vi "运维调试.vi"() -> ()   [LabVIEW 2016]
uses:
  <vilib>/Utility/miscctls.llb/LVPointTypeDef.ctl
  PLC/PLC.lvlib
  <vilib>/Utility/config.llb/NI_LVConfig.lvlib
panel:
  in  "运维调试菜单":T1(xcontrol)
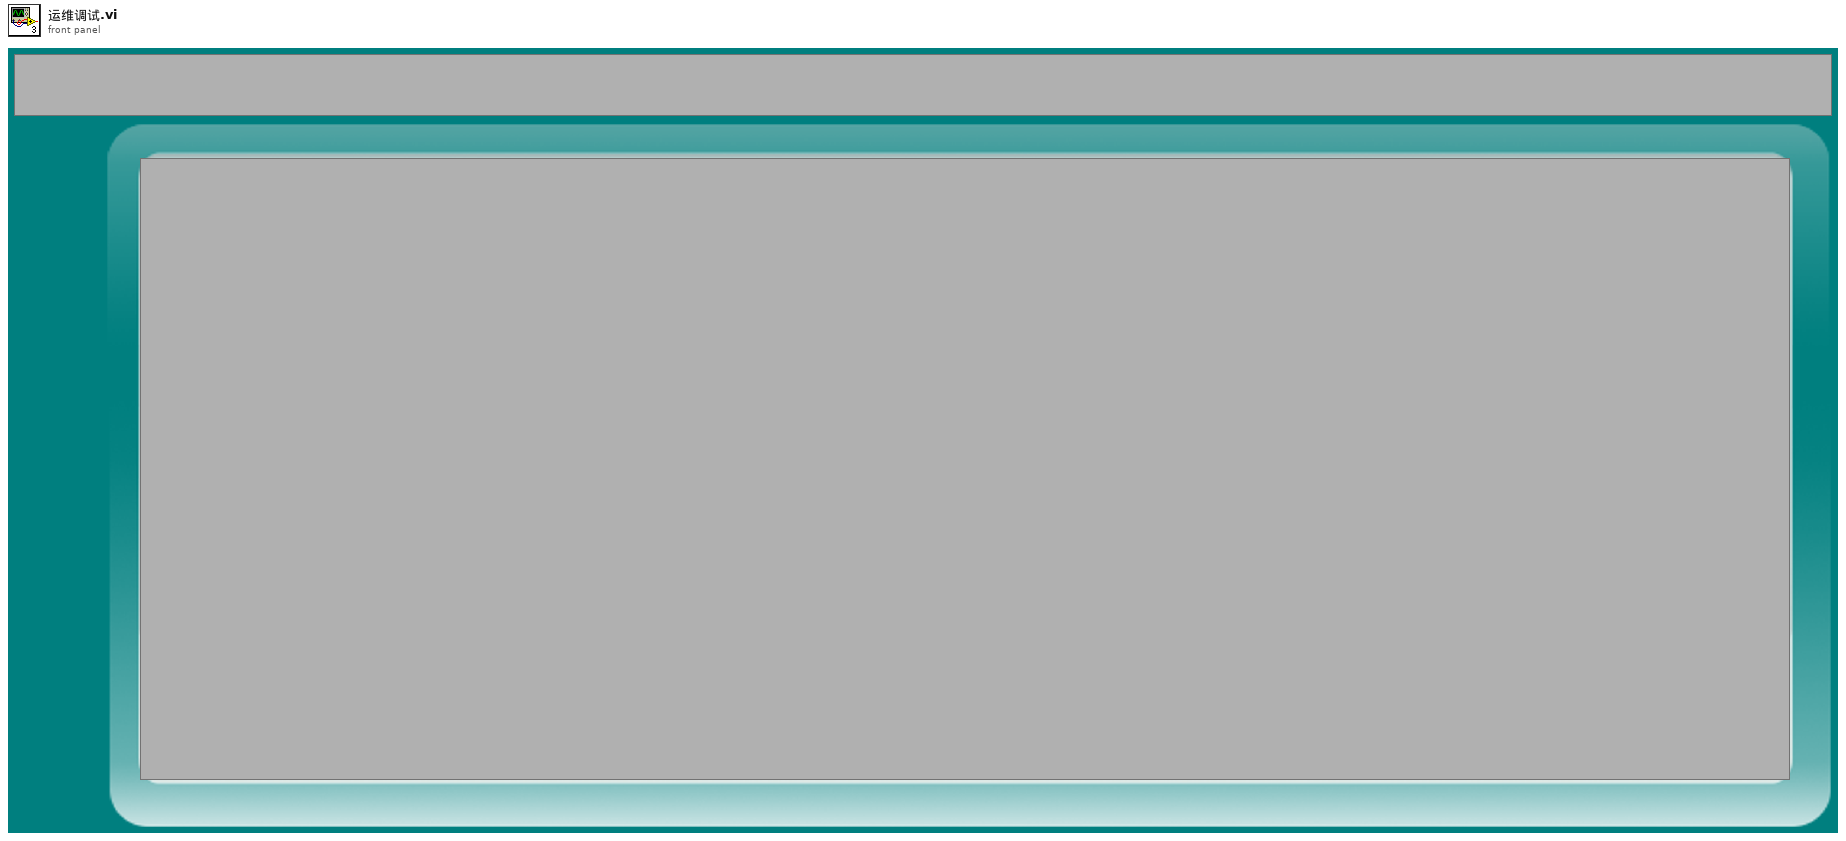
[diagram p1: front panel]
types:
  T1 = enum16{"电源管理", "采配水", "氨氮", "总磷", "总氮", "多参数", "CODMn", "CODcr", "流量计", "质控单元", "超标留样", "其他"}
  T2 = typedef "NI_LVConfig.lvlib/Config Data RefNum.ctl" = refnum<k1>
  T3 = typedef "LVPointTypeDef.ctl" = cluster{"Horizontal":i16, "Vertical":i16}
  T4 = enum16{"Enabled", "Disabled", "Disabled and Grayed Out"}
  T5 = enum32{"Bad", "Idle", "Run top level", "Running"}
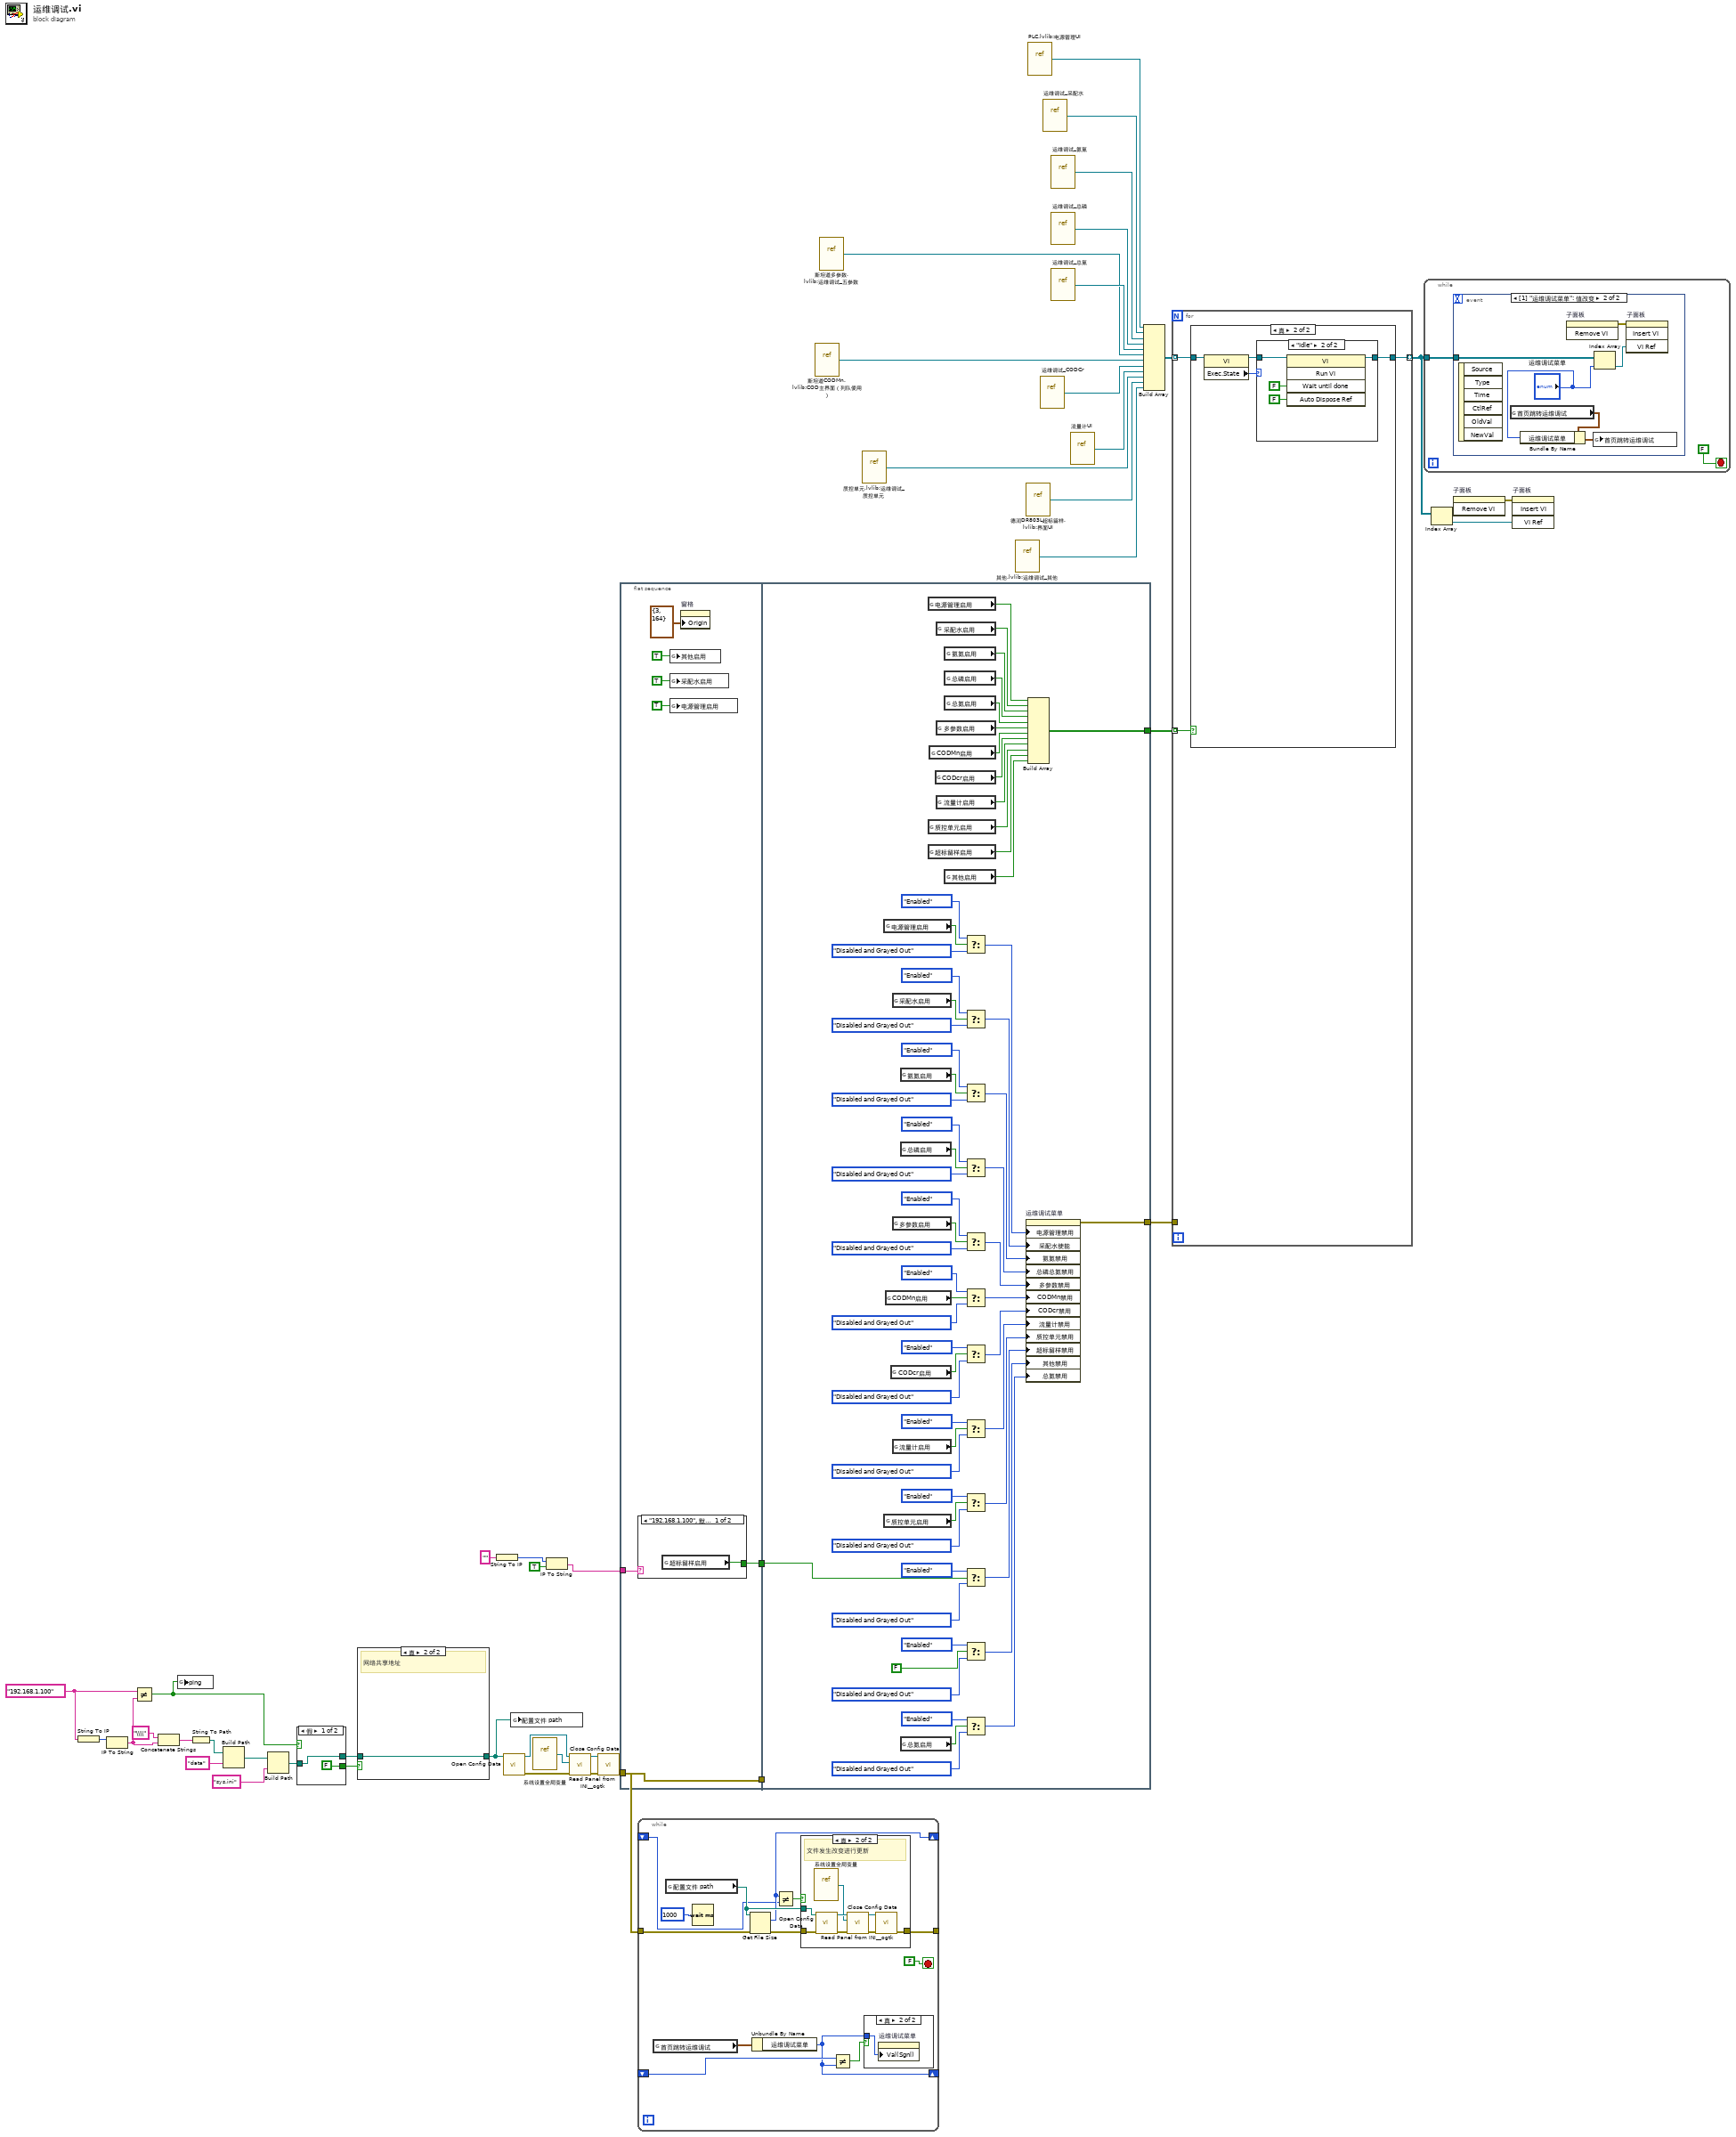
[diagram p0: block diagram]
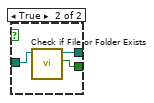
[diagram p4: hidden frame]
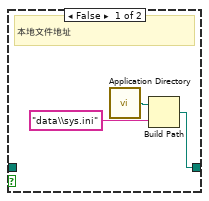
[diagram p5: hidden frame]
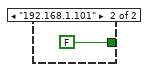
[diagram p6: hidden frame]
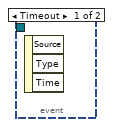
[diagram p9: hidden frame]
diagram:
  w10 = "192.168.1.100" ("名称")
  n1 = String To IP(1:w10) -> (0:w20:u32)
  n2 = IP To String(2:w20) -> (0:w14:string)  [unwired: 1 in]
  n3 = Not Equal?(x=w10, y=w14) -> (x != y?=w8:bool)
  n4 = Concatenate Strings("\\\\" ("字符串"), w14) -> (w17:string)
  n5 = global write "ping全局.vi" "ping"(w8) -> ()
  n6 = String To Path(string=w17) -> (path=w19:path)
  n7 = Build Path(base path=w19, name or relative path="data" ("名称或相对路径")) -> (appended path=w15:path)
  n8 = Build Path(base path=w15, name or relative path="sys.ini" ("名称或相对路径")) -> (appended path=w13:path)
  n9 = case shown="假" w8 {
    tunnel: w13 -> [w45 w49]
    tunnel: [w45 w48] -> w12
    tunnel: [FALSE w47] -> w11
    frame False {
    }
    frame True {
      n10 = call <vilib>:"Check if File or Folder Exists.vi"("path"=w49) -> ("file or folder exists?"=w47:bool, "dup path"=w48:path)  [unwired: 8 in, 1 out]
    }
  }
  n11 = case shown="真" w11 {
    tunnel: w12 -> [_ w53]
    tunnel: [w50 w53] -> w7
    frame False {
      # "本地文件地址"
      n12 = call <vilib>:"Application Directory.vi"() -> ("Application Directory"=w51:path)
      n13 = Build Path(base path=w51, name or relative path="data\\sys.ini" ("名称或相对路径")) -> (appended path=w50:path)
    }
    frame True {
      # "网络共享地址"
    }
  }
  n14 = String To IP(1:"" ("名称")) -> (0:w5:u32)
  n15 = call <vilib>:"Open Config Data.vi"("configuration file path"=w7) -> ("error out"=w35:errorcluster, "refnum"=w34:T2)  [unwired: 8 in, 1 out]
  n16 = global write "ping全局.vi" "配置文件 path"(w7) -> ()
  n17 = vi-ref "系统设置全局变量.vi"() -> (w33:refnum<vi>)
  n18 = IP To String(1:TRUE ("句点符号？(F)"), 2:w5) -> (0:w2:string)
  n19 = call <userlib>:"Read Panel from INI__ogtk.vi"("error in (no error)"=w35, "VI ref"=w33, "refnum"=w34) -> ("error out"=w32:errorcluster, "refnum out"=w31:T2)  [unwired: 7 in]
  n20 = call <vilib>:"Close Config Data.vi"("error in (no error)"=w32, "refnum"=w31) -> ("error out"=w6:errorcluster)  [unwired: 8 in, 1 out]
  n21 = flat-sequence {
    tunnel: w6 -> [w60]
    tunnel: [w60] -> w30
    tunnel: w2 -> [w55]
    tunnel: [w54] -> w1
    tunnel: [w107] -> w36
    tunnel: w30 -> [_]
    tunnel: [w103] -> w29
    tunnel: w1 -> [w64]
    frame #0 {
      n22 = case shown="\"192.168.1.100\", 默认" w55 {
        tunnel: [w61 FALSE] -> w54
        frame "192.168.1.100", Default {
          n23 = global read "系统设置全局变量.vi" "超标留样启用"() -> (w61:bool)
        }
        frame "192.168.1.101" {
        }
      }
      n24 = global write "系统设置全局变量.vi" "其他启用"(TRUE ("其他启用")) -> ()
      n25 = global write "系统设置全局变量.vi" "采配水启用"(TRUE ("采配水启用")) -> ()
      n26 = global write "系统设置全局变量.vi" "电源管理启用"(TRUE ("电源管理启用")) -> ()
      n27 = property on="窗格" class="Pane"("Origin"=T3 {"Horizontal"=3, "Vertical"=164} ("原点")) -> ()  [unwired: 2 in, 2 out]
    }
    frame #1 {
      n28 = global read "系统设置全局变量.vi" "电源管理启用"() -> (w124:bool)
      n29 = global read "系统设置全局变量.vi" "质控单元启用"() -> (w112:bool)
      n30 = global read "系统设置全局变量.vi" "CODMn启用"() -> (w115:bool)
      n31 = global read "系统设置全局变量.vi" "CODcr启用"() -> (w114:bool)
      n32 = global read "系统设置全局变量.vi" "采配水启用"() -> (w121:bool)
      n33 = global read "系统设置全局变量.vi" "多参数启用"() -> (w117:bool)
      n34 = global read "系统设置全局变量.vi" "流量计启用"() -> (w113:bool)
      n35 = global read "系统设置全局变量.vi" "氨氮启用"() -> (w120:bool)
      n36 = global read "系统设置全局变量.vi" "总磷启用"() -> (w65:bool)
      n37 = global read "系统设置全局变量.vi" "总氮启用"() -> (w67:bool)
      n38 = global read "系统设置全局变量.vi" "电源管理启用"() -> (w104:bool)
      n39 = global read "系统设置全局变量.vi" "质控单元启用"() -> (w72:bool)
      n40 = global read "系统设置全局变量.vi" "超标留样启用"() -> (w71:bool)
      n41 = global read "系统设置全局变量.vi" "CODMn启用"() -> (w75:bool)
      n42 = global read "系统设置全局变量.vi" "CODcr启用"() -> (w74:bool)
      n43 = global read "系统设置全局变量.vi" "采配水启用"() -> (w105:bool)
      n44 = global read "系统设置全局变量.vi" "多参数启用"() -> (w76:bool)
      n45 = global read "系统设置全局变量.vi" "流量计启用"() -> (w73:bool)
      n46 = global read "系统设置全局变量.vi" "氨氮启用"() -> (w106:bool)
      n47 = global read "系统设置全局变量.vi" "总磷启用"() -> (w78:bool)
      n48 = global read "系统设置全局变量.vi" "总氮启用"() -> (w77:bool)
      n49 = global read "系统设置全局变量.vi" "其他启用"() -> (w70:bool)
      n50 = Select(t=T4."Enabled" ("电源管理禁用"), s=w124, f=T4."Disabled and Grayed Out" ("电源管理禁用")) -> (s? t:f=w123:T4)
      n51 = Select(t=T4."Enabled" ("电源管理禁用"), s=w121, f=T4."Disabled and Grayed Out" ("电源管理禁用")) -> (s? t:f=w122:T4)
      n52 = Select(t=T4."Enabled" ("电源管理禁用"), s=w120, f=T4."Disabled and Grayed Out" ("电源管理禁用")) -> (s? t:f=w119:T4)
      n53 = Select(t=T4."Enabled" ("电源管理禁用"), s=w65, f=T4."Disabled and Grayed Out" ("电源管理禁用")) -> (s? t:f=w118:T4)
      n54 = Select(t=T4."Enabled" ("电源管理禁用"), s=w117, f=T4."Disabled and Grayed Out" ("电源管理禁用")) -> (s? t:f=w116:T4)
      n55 = Select(t=T4."Enabled" ("电源管理禁用"), s=w115, f=T4."Disabled and Grayed Out" ("电源管理禁用")) -> (s? t:f=w111:T4)
      n56 = Select(t=T4."Enabled" ("电源管理禁用"), s=w114, f=T4."Disabled and Grayed Out" ("电源管理禁用")) -> (s? t:f=w110:T4)
      n57 = Select(t=T4."Enabled" ("电源管理禁用"), s=w113, f=T4."Disabled and Grayed Out" ("电源管理禁用")) -> (s? t:f=w109:T4)
      n58 = Select(t=T4."Enabled" ("电源管理禁用"), s=w112, f=T4."Disabled and Grayed Out" ("电源管理禁用")) -> (s? t:f=w108:T4)
      n59 = Select(t=T4."Enabled" ("电源管理禁用"), s=w64, f=T4."Disabled and Grayed Out" ("电源管理禁用")) -> (s? t:f=w79:T4)
      n60 = Select(t=T4."Enabled" ("电源管理禁用"), s=FALSE, f=T4."Disabled and Grayed Out" ("电源管理禁用")) -> (s? t:f=w82:T4)
      n61 = Select(t=T4."Enabled" ("电源管理禁用"), s=w67, f=T4."Disabled and Grayed Out" ("电源管理禁用")) -> (s? t:f=w66:T4)
      n62 = property on="运维调试菜单" class="运维调试菜单 (严格)"("电源管理禁用"=w123, "采配水使能"=w122, "氨氮禁用"=w119, "总磷总氮禁用"=w118, "多参数禁用"=w116, "CODMn禁用"=w111, "CODcr禁用"=w110, "流量计禁用"=w109, "质控单元禁用"=w108, "超标留样禁用"=w79, "其他禁用"=w82, "总氮禁用"=w66) -> (error out=w107:errorcluster)  [unwired: 2 in, 1 out]
      n63 = Build Array(w104, w105, w106, w78, w77, w76, w75, w74, w73, w72, w71, w70) -> (w103:bool[])
    }
  }
  n64 = while {
    tunnel: w6 -> [w133]
    tunnel: [w136] -> _
    shift-right: [w132] -> _
    shift-left: _ -> [w131]
    shift-right: [w125] -> _
    shift-left: _ -> [w127]
    stop <- FALSE stop-if-true
    n65 = global read "系统设置全局变量.vi" "首页跳转运维调试"() -> (w128:cluster{"主画面菜单":i32, "运维调试菜单":i32})
    n66 = global read "ping全局.vi" "配置文件 path"() -> (w134:path)
    n67 = Wait (ms)(milliseconds to wait=u32 1000 ("等待时间（毫秒）")) -> ()  [unwired: 1 out]
    n68 = Get File Size(file=w134, error in=w133) -> (size (in bytes)=w132:i64, 0:w129:errorcluster)  [unwired: 1 out]
    n69 = Unbundle By Name(w128) -> ("运维调试菜单"=w125:i32)
    n70 = Not Equal?(x=w132, y=w131) -> (x != y?=w130:bool)
    n71 = case shown="真" w130 {
      tunnel: [w139 w142] -> w136
      tunnel: w134 -> [_ w141]
      tunnel: w129 -> [w139 w140]
      frame False {
      }
      frame True {
        # "文件发生改变进行更新"
        n72 = vi-ref "系统设置全局变量.vi"() -> (w145:refnum<vi>)
        n73 = call <vilib>:"Open Config Data.vi"("error in (no error)"=w140, "configuration file path"=w141) -> ("error out"=w147:errorcluster, "refnum"=w146:T2)  [unwired: 7 in, 1 out]
        n74 = call <userlib>:"Read Panel from INI__ogtk.vi"("error in (no error)"=w147, "VI ref"=w145, "refnum"=w146) -> ("error out"=w144:errorcluster, "refnum out"=w143:T2)  [unwired: 7 in]
        n75 = call <vilib>:"Close Config Data.vi"("error in (no error)"=w144, "refnum"=w143) -> ("error out"=w142:errorcluster)  [unwired: 8 in, 1 out]
      }
    }
    n76 = Not Equal?(x=w127, y=w125) -> (x != y?=w126:bool)
    n77 = case shown="真" w126 {
      tunnel: w125 -> [_ w138]
      frame False {
      }
      frame True {
        n78 = property on="运维调试菜单" class="运维调试菜单 (严格)"("Val(Sgnl)"=w138) -> ()  [unwired: 2 in, 2 out]
      }
    }
  }
  n79 = vi-ref "斯坦道CODMn.lvlib:COD主界面（列队使用）.vi"() -> (w26:refnum<vi>)
  n80 = vi-ref "斯坦道多参数.lvlib:运维调试_五参数.vi"() -> (w27:refnum<vi>)
  n81 = vi-ref "质控单元.lvlib:运维调试_质控单元.vi"() -> (w23:refnum<vi>)
  n82 = vi-ref "其他.lvlib:运维调试_其他.vi"() -> (w21:refnum<vi>)
  n83 = vi-ref "德润DR803L超标留样.lvlib:界面UI.vi"() -> (w22:refnum<vi>)
  n84 = vi-ref "PLC.lvlib:电源管理UI.vi"() -> (w37:refnum<vi>)
  n85 = vi-ref "运维调试_CODCr.vi"() -> (w25:refnum<vi>)
  n86 = vi-ref "运维调试_采配水.vi"() -> (w40:refnum<vi>)
  n87 = vi-ref "运维调试_氨氮.vi"() -> (w39:refnum<vi>)
  n88 = vi-ref "运维调试_总磷.vi"() -> (w38:refnum<vi>)
  n89 = vi-ref "运维调试_总氮.vi"() -> (w28:refnum<vi>)
  n90 = vi-ref "流量计UI.vi"() -> (w24:refnum<vi>)
  n91 = Build Array(w37, w40, w39, w38, w28, w27, w26, w25, w24, w23, w22, w21) -> (w41:refnum<vi>[])
  n92 = for {
    tunnel: w41 -> [w150] mode=indexing
    tunnel: [w149] -> w43 mode=indexing
    tunnel: w29 -> [w148] mode=indexing
    tunnel: w36 -> [_]
    n93 = case shown="真" w148 {
      tunnel: w150 -> [w151 w155]
      tunnel: [w151 w152] -> w149
      frame False {
      }
      frame True {
        n94 = property class="VI"(reference=w155) -> (reference out=w153:refnum<vi>, "Exec.State"=w154:T5)  [unwired: 1 in, 1 out]
        n95 = case shown="\"Idle\"" w154 {
          tunnel: w153 -> [w156 w158]
          tunnel: [w156 w157] -> w152
          frame "Bad", Default {
          }
          frame "Idle" {
            n96 = invoke class="VI" method="Run VI"(reference=w158, "Wait until done"=FALSE ("结束前等待"), "Auto Dispose Ref"=FALSE ("自动销毁引用")) -> (reference out=w157:refnum<vi>)  [unwired: 2 in, 4 out]
          }
        }
      }
    }
  }
  n97 = while {
    tunnel: w43 -> [w161]
    stop <- FALSE stop-if-true
    n98 = event shown="[1] \"运维调试菜单\": 值改变" {
      selector: _ -> [_ _]
      dyn-events: _ -> [_ _]
      timeout: _ -> [_ _]
      tunnel: w161 -> [_ w167]
      event Timeout {
        n99 = event-data() -> ()  [unwired: 1 in, 3 out]
      }
      event "运维调试菜单": Value Change {
        n100 = event-data() -> ()  [unwired: 1 in, 6 out]
        n101 = global read "系统设置全局变量.vi" "首页跳转运维调试"() -> (w165:cluster{"主画面菜单":i32, "运维调试菜单":i32})
        n102 = Bundle By Name(cluster=w165, "运维调试菜单"="运维调试菜单") -> (w164:cluster{"主画面菜单":i32, "运维调试菜单":i32})
        n103 = invoke on="子面板" class="SubPnl" method="Remove VI"() -> (error out=w168:errorcluster)  [unwired: 3 in, 2 out]
        n104 = global write "系统设置全局变量.vi" "首页跳转运维调试"(w164) -> ()
        n105 = Index Array(array=w167, index="运维调试菜单") -> (element=w166:refnum<vi>)
        n106 = invoke on="子面板" class="SubPnl" method="Insert VI"(error in=w168, "VI Ref"=w166) -> ()  [unwired: 2 in, 4 out]
      }
    }
  }
  n107 = Index Array(array=w43) -> (element=w42:refnum<vi>)  [unwired: 1 in]
  n108 = invoke on="子面板" class="SubPnl" method="Remove VI"() -> (error out=w44:errorcluster)  [unwired: 3 in, 2 out]
  n109 = invoke on="子面板" class="SubPnl" method="Insert VI"(error in=w44, "VI Ref"=w42) -> ()  [unwired: 2 in, 4 out]
